vi "ALTS-2015 Get Sensor Name.vi"(8 "error in (no error)":errorcluster, 11 "Station Enum":T1) -> (0 "error out":errorcluster, 3 "Sensor Name":string)   [LabVIEW 2013]
doc: "Copyright © 2005, Soliton Technologies.\nAll rights reserved."
uses:
  Controls/ALTS-2015 Station Cluster.ctl
  Controls/ALTS-2015 LV2GBL Options.ctl
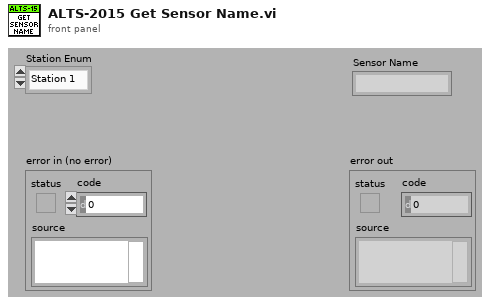
[diagram p1: front panel]
types:
  T1 = typedef "ALTS-2015 Station Cluster.ctl" = enum16{"Station 1", "Station 2", "Station 3", "Station 4"}
  T2 = typedef "ALTS-2015 LV2GBL Options.ctl" = enum16{"Read all", "Write all"}
  T3 = typedef "ALTS-2015 INI Configuration Cluster.ctl" = cluster{"Application":cluster{"Rerun Count":i32, "Workorder No":string, "PLC Scanner":bool}, "Station Details":cluster{"Sensor Name 1":string, "Sensor Name 2":string, "Sensor Name 3":string, "Sensor Name 4":string, "Station1 Enable":bool, "Station2 Enable":bool, "Station3 Enable":bool, "Station4 Enable":bool}, "Database":cluster{"Database Connection Link":path, "Result Procedure":string, "User":string, "Password":string, "Prompt":bool, "Station 1 LT Result DB DSN Path":path, "Station 2 LT Result DB DSN Path":path, "Station 3 LT Result DB DSN Path":path, "Station 4 LT Result DB DSN Path":path, "AirLeakTestResult Procedure":string, "Serial Details Procedure":string}, "Simulation":cluster{"Simulate DAQ Hardware":bool, "Simulate Result DB Write":bool, "Simulate Scanner":bool, "Simulate OPC":bool, "Simulate Serial Details DB":bool, "Simulate Result DB":bool, "Simulate Scanner DB Path":path, "Simulate Serial Details DB Path":path, "Simulate Result DB Path":path}, "Barcode Scanner1":cluster{"Scanner IP":string, "Scanner Port":u16, "#Bytes to Read":i32, "Timeout_ms":i32}, "Barcode Scanner2":cluster{"Enabled?":bool, "Scanner IP":string, "Scanner Port":u16, "#Bytes to Read":i32}}
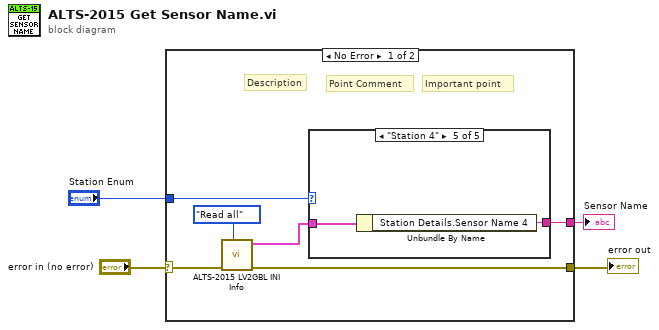
[diagram p0: block diagram]
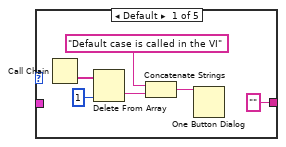
[diagram p2: hidden frame]
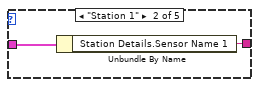
[diagram p3: hidden frame]
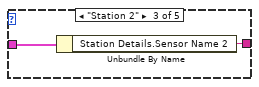
[diagram p4: hidden frame]
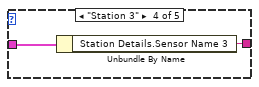
[diagram p5: hidden frame]
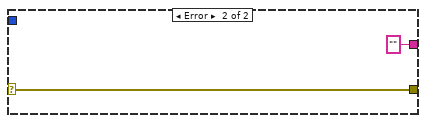
[diagram p6: hidden frame]
diagram:
  n1 = case shown="No Error" "error in (no error)" {
    selector: "error in (no error)" -> [w8 w26]
    tunnel: [w10 w26] -> w3
    tunnel: "Station Enum" -> [w6 _]
    tunnel: [w5 "" ("Sensor Name 4")] -> w1
    frame No Error {
      # "Point Comment"
      # "Important point"
      # "Description"
      n2 = call "ALTS-2015 LV2GBL INI Info.vi"("Options"=ALTS-2015_LV2GBL_Options."Read all", "error in"=w8) -> ("error out"=w10:errorcluster, "Configuration Cluster Out"=w7:T3)  [unwired: 8 in]
      n3 = case shown="\"Station 4\"" w6 {
        tunnel: w7 -> [_ w18 w20 w22 w24]
        tunnel: ["" ("Sensor Name 4") w17 w19 w21 w23] -> w5
        frame Default {
          n4 = Call Chain() -> (call chain=w12:string[])
          n5 = Delete From Array(array=w12, index=1) -> (deleted portion=w11:string)  [unwired: 1 in, 1 out]
          n6 = Concatenate Strings("Default case is called in the VI" ("message"), w11) -> (w14:string)
          n7 = One Button Dialog(message=w14) -> ()  [unwired: 1 in, 1 out]
        }
        frame "Station 1" {
          n8 = Unbundle By Name(w18) -> ("Station Details.Sensor Name 1"=w17:string)
        }
        frame "Station 2" {
          n9 = Unbundle By Name(w20) -> ("Station Details.Sensor Name 2"=w19:string)
        }
        frame "Station 3" {
          n10 = Unbundle By Name(w22) -> ("Station Details.Sensor Name 3"=w21:string)
        }
        frame "Station 4" {
          n11 = Unbundle By Name(w24) -> ("Station Details.Sensor Name 4"=w23:string)
        }
      }
    }
    frame Error {
    }
  }
  "error out" <- w3
  "Sensor Name" <- w1
